vi "formatMotorsToString.vi"(0 "Light 3":i32, 1 "Light 2":i32, 2 "zone 3 inlet":dbl, 3 "Light 1":i32, 4 "zone 3 co2":dbl, 5 "error in (no error)":errorcluster, 6 "zone 2 return":dbl, 7 "fresh air":dbl, 8 "zone 2 inlet":dbl, 9 "zone 2 co2":dbl, 10 "zone 1 return":dbl, 11 "zone 1 co2":dbl, 12 "zone 1 inlet":dbl, 13 "zone 3 return":dbl) -> (14 "String":string, 19 "error out":errorcluster)   [LabVIEW 2019]
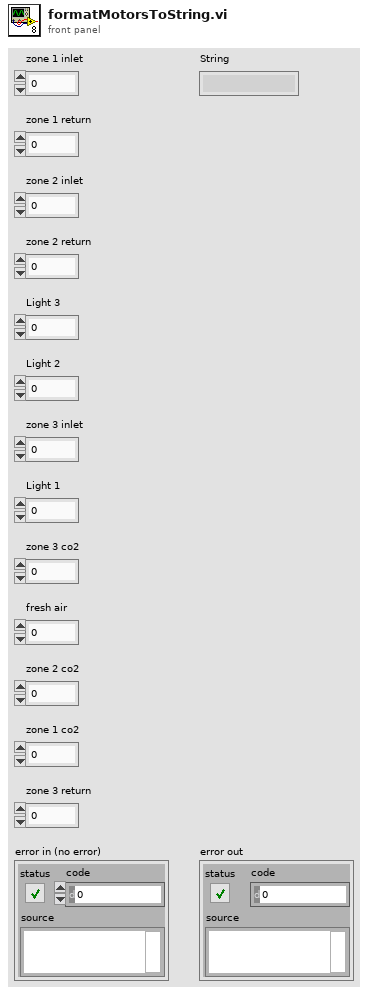
[diagram p1: front panel]
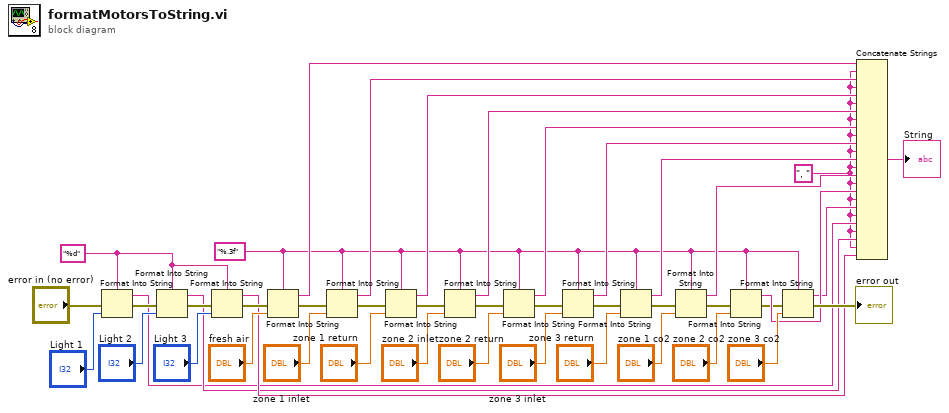
[diagram p0: block diagram]
diagram:
  w5 = "%d" ("format string")
  w9 = "%.3f" ("format string")
  w1 = ", "
  n1 = Format Into String(format string=w5, error in="error in (no error)", "Light 1") -> (resulting string=w2:string, error out=w8:errorcluster)  [unwired: 1 in]
  n2 = Format Into String(format string=w5, error in=w8, "Light 2") -> (resulting string=w3:string, error out=w7:errorcluster)  [unwired: 1 in]
  n3 = Format Into String(format string=w5, error in=w7, "Light 3") -> (resulting string=w4:string, error out=w6:errorcluster)  [unwired: 1 in]
  n4 = Format Into String(format string=w9, error in=w6, "fresh air") -> (resulting string=w28:string, error out=w18:errorcluster)  [unwired: 1 in]
  n5 = Format Into String(format string=w9, error in=w18, "zone 1 inlet") -> (resulting string=w27:string, error out=w17:errorcluster)  [unwired: 1 in]
  n6 = Format Into String(format string=w9, error in=w17, "zone 1 return") -> (resulting string=w26:string, error out=w16:errorcluster)  [unwired: 1 in]
  n7 = Format Into String(format string=w9, error in=w16, "zone 2 inlet") -> (resulting string=w25:string, error out=w15:errorcluster)  [unwired: 1 in]
  n8 = Format Into String(format string=w9, error in=w15, "zone 2 return") -> (resulting string=w24:string, error out=w14:errorcluster)  [unwired: 1 in]
  n9 = Format Into String(format string=w9, error in=w14, "zone 3 inlet") -> (resulting string=w23:string, error out=w13:errorcluster)  [unwired: 1 in]
  n10 = Format Into String(format string=w9, error in=w13, "zone 3 return") -> (resulting string=w22:string, error out=w12:errorcluster)  [unwired: 1 in]
  n11 = Format Into String(format string=w9, error in=w12, "zone 1 co2") -> (resulting string=w21:string, error out=w11:errorcluster)  [unwired: 1 in]
  n12 = Format Into String(format string=w9, error in=w11, "zone 2 co2") -> (resulting string=w20:string, error out=w10:errorcluster)  [unwired: 1 in]
  n13 = Format Into String(format string=w9, error in=w10, "zone 3 co2") -> (resulting string=w19:string, error out=→"error out":errorcluster)  [unwired: 1 in]
  n14 = Concatenate Strings(w28, w1, w27, w1, w26, w1, w25, w1, w24, w1, w23, w1, w22, w1, w21, w1, w20, w1, w19, w1, w2, w1, w3, w1, w4) -> (→"String":string)
